vi "Edit-measurement-settings.vi"(8 "error in (no error)":errorcluster, 11 "Object ref in":T1) -> (0 "error out":errorcluster, 3 "Object ref out":T1)   [LabVIEW 2013, in "MaterialCharacterization.lvlib" / "MC-Main.lvclass"]
uses:
  MC-Main.lvclass
  Object-reference.ctl
  MC-Main.lvclass/MC-Main.ctl
  Read Measurement type.vi
  Read Parser.vi
  Read SM1000.vi
  ScanParser/MC-ScanParser.lvclass
  SM1000/MC-SM1000.lvclass
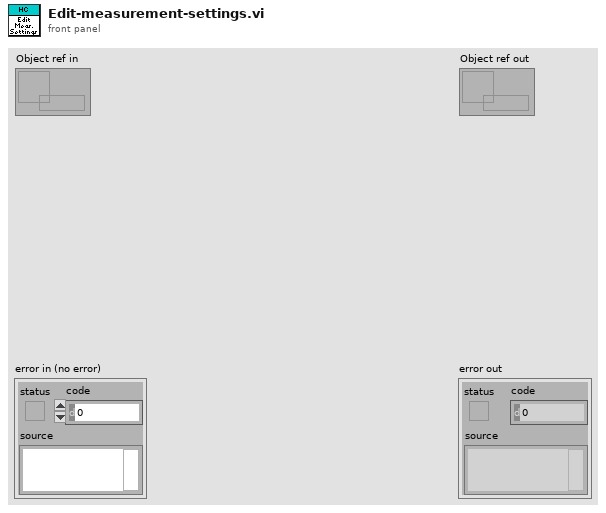
[diagram p1: front panel]
types:
  T1 = typedef "MaterialCharacterization.lvlib/MC-Main.lvclass/Object-reference.ctl" = refnum<data-value>
  T2 = typedef "MaterialCharacterization.lvlib/MC-Main.lvclass/Measurement-types.ctl" = enum16{"Scan file analysis", "Thermal conductivity", "Laser reflection", "Combined"}
  T3 = typedef "MaterialCharacterization.lvlib/MC-ScanParser.lvclass/Object-reference.ctl" = refnum<data-value>
  T4 = typedef "MaterialCharacterization.lvlib/MC-SM1000.lvclass/Object-reference.ctl" = refnum<data-value>
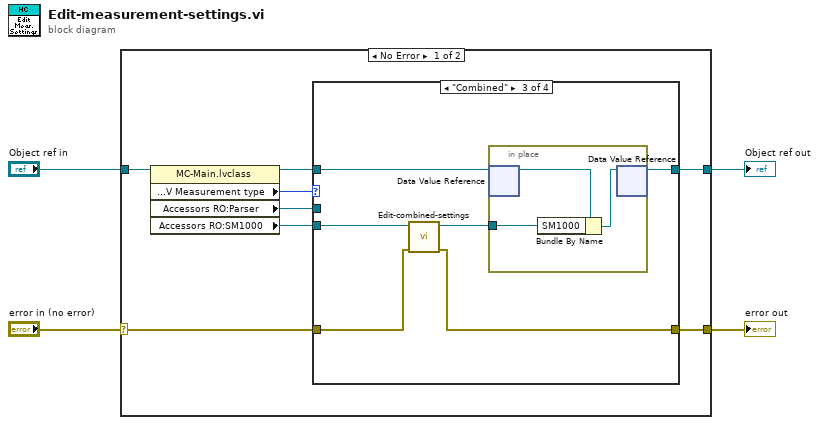
[diagram p0: block diagram]
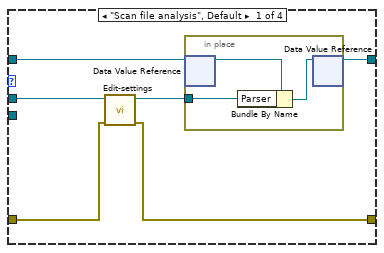
[diagram p2: hidden frame]
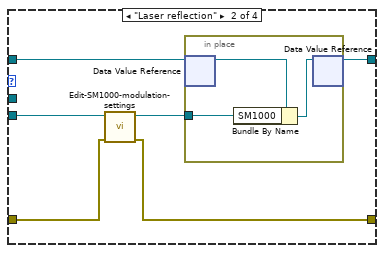
[diagram p3: hidden frame]
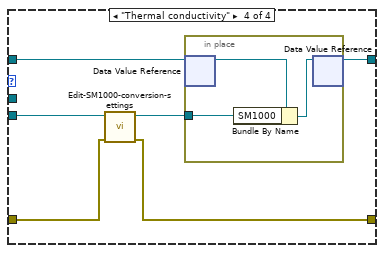
[diagram p4: hidden frame]
diagram:
  n1 = case shown="No Error" "error in (no error)" {
    selector: "error in (no error)" -> [w8 w50]
    tunnel: [w7 w50] -> w3
    tunnel: [w9 w49] -> w1
    tunnel: "Object ref in" -> [w12 w49]
    frame No Error {
      n2 = property class="MC-Main.lvclass"(reference=w12) -> (reference out=w10:T1, "Accessors/Modifiers:V Measurement type"=w11:T2, "Accessors RO:Parser"=w6:T3, "Accessors RO:SM1000"=w5:T4)  [unwired: 1 in, 1 out]
      n3 = case shown="\"Combined\"" w11 {
        tunnel: w10 -> [w17 w27 w36 w45]
        tunnel: [w16 w26 w35 w44] -> w9
        tunnel: w8 -> [w14 w24 w32 w42]
        tunnel: [w13 w23 w31 w41] -> w7
        tunnel: w6 -> [w18 _ _ _]
        tunnel: w5 -> [_ w22 w33 w40]
        frame "Scan file analysis", Default {
          n4 = call "Edit-settings.vi"("error in (no error)"=w14, "Reference in"=w18) -> ("error out"=w13:errorcluster, "Reference out"=w15:T3)  [unwired: 8 in]
          n5 = in-place {
            in-place-border: w15 -> [w19]
            n6 = in-place-dvr #1(w17) -> (w21:refnum<class "MC-Main.lvclass">)  [unwired: 1 out]
            n7 = Bundle By Name(cluster=w21, "Parser"=w19) -> (w20:refnum<class "MC-Main.lvclass">)
            n8 = in-place-dvr #1(w20) -> (w16:T1)  [unwired: 1 out]
          }
        }
        frame "Laser reflection" {
          n9 = call "Edit-SM1000-modulation-settings.vi"("error in (no error)"=w24, "Reference in"=w22) -> ("error out"=w23:errorcluster, "Reference out"=w25:T4)  [unwired: 8 in]
          n10 = in-place {
            in-place-border: w25 -> [w28]
            n11 = in-place-dvr #2(w27) -> (w30:refnum<class "MC-Main.lvclass">)  [unwired: 1 out]
            n12 = Bundle By Name(cluster=w30, "SM1000"=w28) -> (w29:refnum<class "MC-Main.lvclass">)
            n13 = in-place-dvr #2(w29) -> (w26:T1)  [unwired: 1 out]
          }
        }
        frame "Combined" {
          n14 = call "Edit-combined-settings.vi"("error in (no error)"=w32, "Reference in"=w33) -> ("error out"=w31:errorcluster, "Reference out"=w34:T4)  [unwired: 8 in]
          n15 = in-place {
            in-place-border: w34 -> [w37]
            n16 = in-place-dvr #3(w36) -> (w39:refnum<class "MC-Main.lvclass">)  [unwired: 1 out]
            n17 = Bundle By Name(cluster=w39, "SM1000"=w37) -> (w38:refnum<class "MC-Main.lvclass">)
            n18 = in-place-dvr #3(w38) -> (w35:T1)  [unwired: 1 out]
          }
        }
        frame "Thermal conductivity" {
          n19 = call "Edit-SM1000-conversion-settings.vi"("error in (no error)"=w42, "Reference in"=w40) -> ("error out"=w41:errorcluster, "Reference out"=w43:T4)  [unwired: 8 in]
          n20 = in-place {
            in-place-border: w43 -> [w46]
            n21 = in-place-dvr #4(w45) -> (w48:refnum<class "MC-Main.lvclass">)  [unwired: 1 out]
            n22 = Bundle By Name(cluster=w48, "SM1000"=w46) -> (w47:refnum<class "MC-Main.lvclass">)
            n23 = in-place-dvr #4(w47) -> (w44:T1)  [unwired: 1 out]
          }
        }
      }
    }
    frame Error {
    }
  }
  "error out" <- w3
  "Object ref out" <- w1
